vi "Turn channels off (subVI).vi"() -> (3 "String":string)   [LabVIEW 2018]
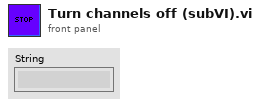
[diagram p1: front panel]
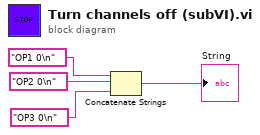
[diagram p0: block diagram]
diagram:
  n1 = Concatenate Strings("OP1 0\n", "OP2 0\n", "OP3 0\n") -> (→"String":string)
